vi "ql2_query_build.vi"(9 "options (key,val)":string[][](array[string]), 10 "term":string, 11 "query_type":T1) -> (3 "query":string)   [LabVIEW 2017, in "rethinkdb.lvlib"]
uses:
  rethinkdb.lvlib
  ql2_query.ctl
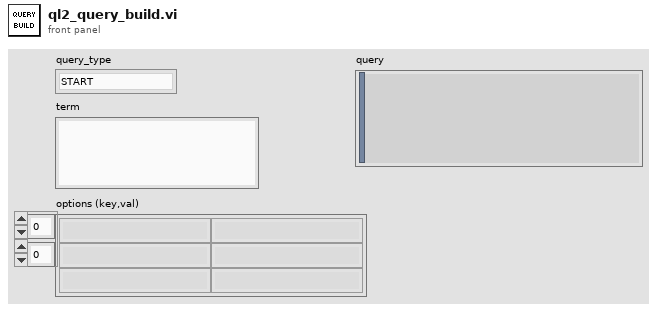
[diagram p1: front panel]
types:
  T1 = typedef "rethinkdb.lvlib/ql2_query.ctl" = enum8{"START", "CONTINUE", "STOP", "NOREPLY_WAIT", "SERVER_INFO", "invalid"}
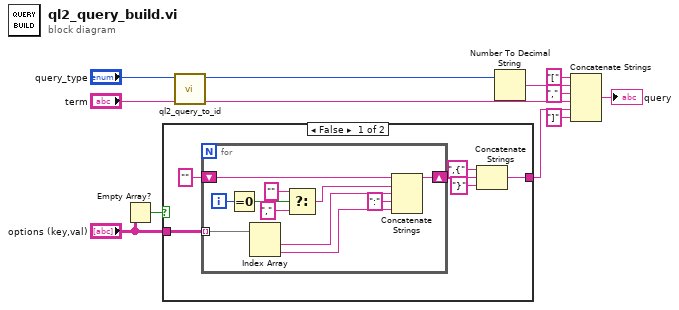
[diagram p0: block diagram]
diagram:
  n1 = Empty Array?(array="options (key,val)") -> (empty?=w4:bool)
  n2 = case shown="False" w4 {
    tunnel: "options (key,val)" -> [w16 _]
    tunnel: [w14 _] -> w6
    frame False {
      n3 = for {
        tunnel: w16 -> [w21] mode=indexing
        shift-right: [w23] -> w15
        shift-left: "" -> [w28]
        i -> [w27]
        n4 = Equal To 0?(x=w27) -> (x = 0?=w26:bool)
        n5 = Index Array(array=w21) -> (element #1=w20:string, element #2=w18:string)  [unwired: 2 in]
        n6 = Select(t="", s=w26, f=",") -> (s? t:f=w22:string)
        n7 = Concatenate Strings(w28, w22, w20, ":" ("string"), w18) -> (w23:string)
      }
      n8 = Concatenate Strings(",{" ("string"), w15, "}" ("string")) -> (w14:string)
    }
    frame True {
    }
  }
  n9 = call "ql2_query_to_id.vi"("query_type"="query_type") -> ("id"=w1:u32)  [unwired: 9 in, 1 out]
  n10 = Number To Decimal String(number=w1) -> (decimal integer string=w11:string)  [unwired: 1 in]
  n11 = Concatenate Strings("[" ("string"), w11, "," ("string"), "term", w6, "]" ("string")) -> (→"query":string)
